vi "Find next channel.vi"(8 "error in (no error)":errorcluster, 11 "Item Ref out in":T1 format="%.0x") -> (0 "error out":errorcluster, 2 "Label out":string, 3 "Item Ref out out":T1 format="%.0x")   [LabVIEW 2017, in "GE_RM_System Explorer.lvlib"]
uses:
  GE_RM_System Explorer.lvlib
  <vilib>/NI Veristand/Custom Device API/Custom Device Item Ref.ctl
  <vilib>/NI Veristand/Custom Device API/Custom Device API.lvlib
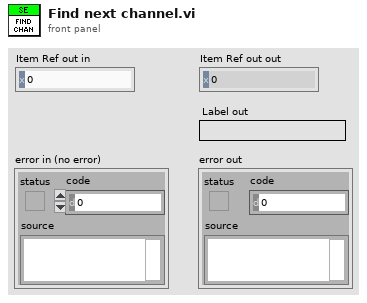
[diagram p1: front panel]
types:
  T1 = typedef "Custom Device API.lvlib/Custom Device Item Ref.ctl" = u64
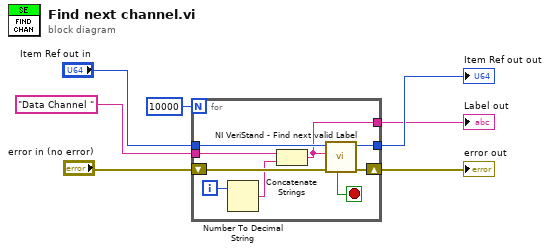
[diagram p0: block diagram]
diagram:
  n1 = for {
    N: 10000 -> [_]
    tunnel: "Data Channel " ("Label") -> [w11]
    tunnel: "Item Ref out in" -> [w15]
    tunnel: [w13] -> w3
    shift-right: [w12] -> w2
    shift-left: "error in (no error)" -> [w16]
    tunnel: [w9] -> w1
    i -> [w10]
    stop <- w14 stop-if-true
    n2 = Number To Decimal String(number=w10) -> (decimal integer string=w8:string)  [unwired: 1 in]
    n3 = Concatenate Strings(w11, w8) -> (w9:string)
    n4 = call <vilib>:"NI VeriStand - Find next valid Label.vi"("error in (no error)"=w16, "Label"=w9, "Item Ref in"=w15) -> ("error out"=w12:errorcluster, "Item Ref out"=w13:T1, "Requested label not in use?"=w14:bool)  [unwired: 4 in, 2 out]
  }
  "error out" <- w2
  "Item Ref out out" <- w3
  "Label out" <- w1
